vi "Write Check Revocation.vi"(8 "error in (no error)":errorcluster, 10 "Check Revocation":bool, 11 "dotNET SSL Server in":refnum<class "dotNET SSL Socket.lvclass">) -> (0 "error out":errorcluster, 3 "dotNET SSL Server out":refnum<class "dotNET SSL Socket.lvclass">)   [LabVIEW 2013, in "dotNET SSL Socket.lvlib" / "dotNET SSL Socket.lvclass"]
uses:
  dotNET SSL Socket.lvclass
  dotNET SSL Socket.lvclass/dotNET SSL Socket.ctl
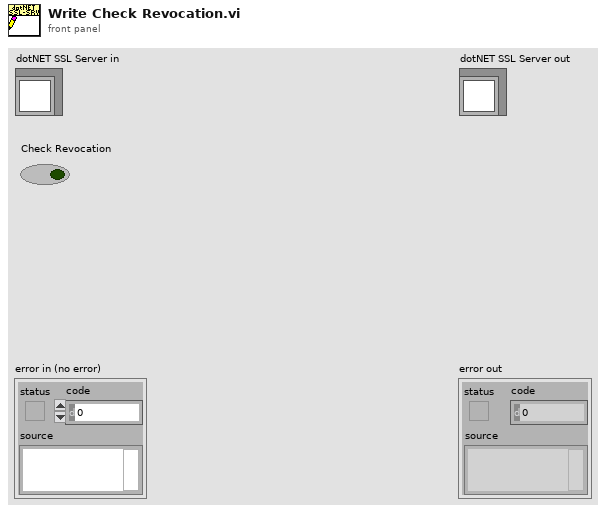
[diagram p1: front panel]
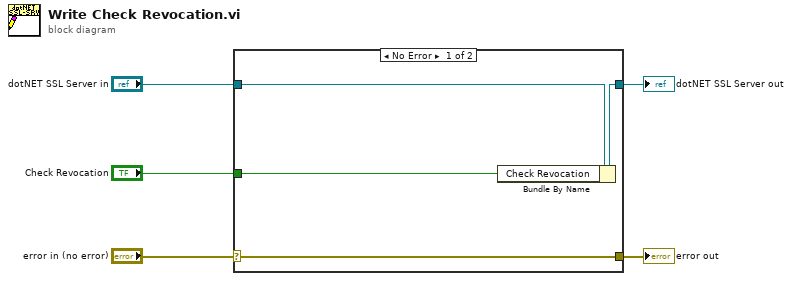
[diagram p0: block diagram]
diagram:
  n1 = case shown="No Error" "error in (no error)" {
    selector: "error in (no error)" -> [w9 w10]
    tunnel: [w9 w10] -> w4
    tunnel: [w7 w11] -> w2
    tunnel: "dotNET SSL Server in" -> [w8 w11]
    tunnel: "Check Revocation" -> [w6 _]
    frame No Error {
      n2 = Bundle By Name(cluster=w8, "Check Revocation"=w6) -> (w7:refnum<class "dotNET SSL Socket.lvclass">)
    }
    frame Error {
    }
  }
  "error out" <- w4
  "dotNET SSL Server out" <- w2
